vi "2 MissionHeadingGoodness.vi"(6 "Waypoint in":refnum<class "Waypoint.lvclass">, 8 "Waypoint Location":T3 {"North" format="%#_10f"; "East" format="%#_8f"}, 9 "Heading\nto Test":T2 format="%05.1f", 10 "UW Tack":dbl, 11 "Into irons?":bool) -> (0 "Pure Waypoint Goodness":dbl, 1 "Direction Change Goodness":dbl, 2 "No-Sail Goodness":dbl, 3 "Target Goodness":dbl, 4 "Pure Wind Goodness":dbl)   [LabVIEW 2011]
doc: "This VI simply takes in a heading to test, runs the necessary component goodness functions and outputs their \"goodness value\" for that heading."
uses:
  2 Typedefs/UTM Location.ctl
  2 Classes/Waypoint/Waypoint.lvclass
  2 Typedefs/heading.ctl
  2 Typedefs/apparent wind direction.ctl
  2 Globals/2 Global.vi
  2 Globals/2 TuningConstants.vi
panel:
  out "Heading Goodness":T1
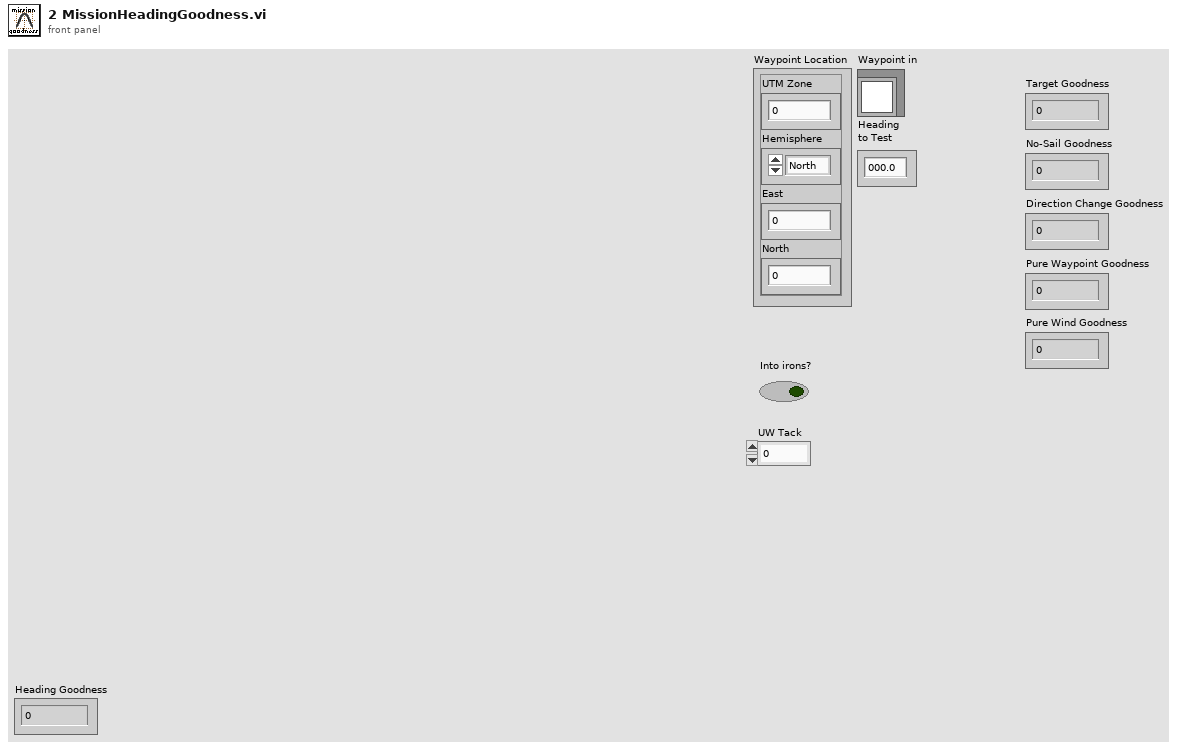
[diagram p1: front panel]
types:
  T1 = typedef "apparent wind direction.ctl" = dbl
  T2 = typedef "heading.ctl" = dbl
  T3 = typedef "UTM Location.ctl" = cluster{"UTM Zone":dbl, "Hemisphere":enum16{"North", "South"}, "East":dbl, "North":dbl}
  T4 = typedef "absolute wind direction.ctl" = dbl
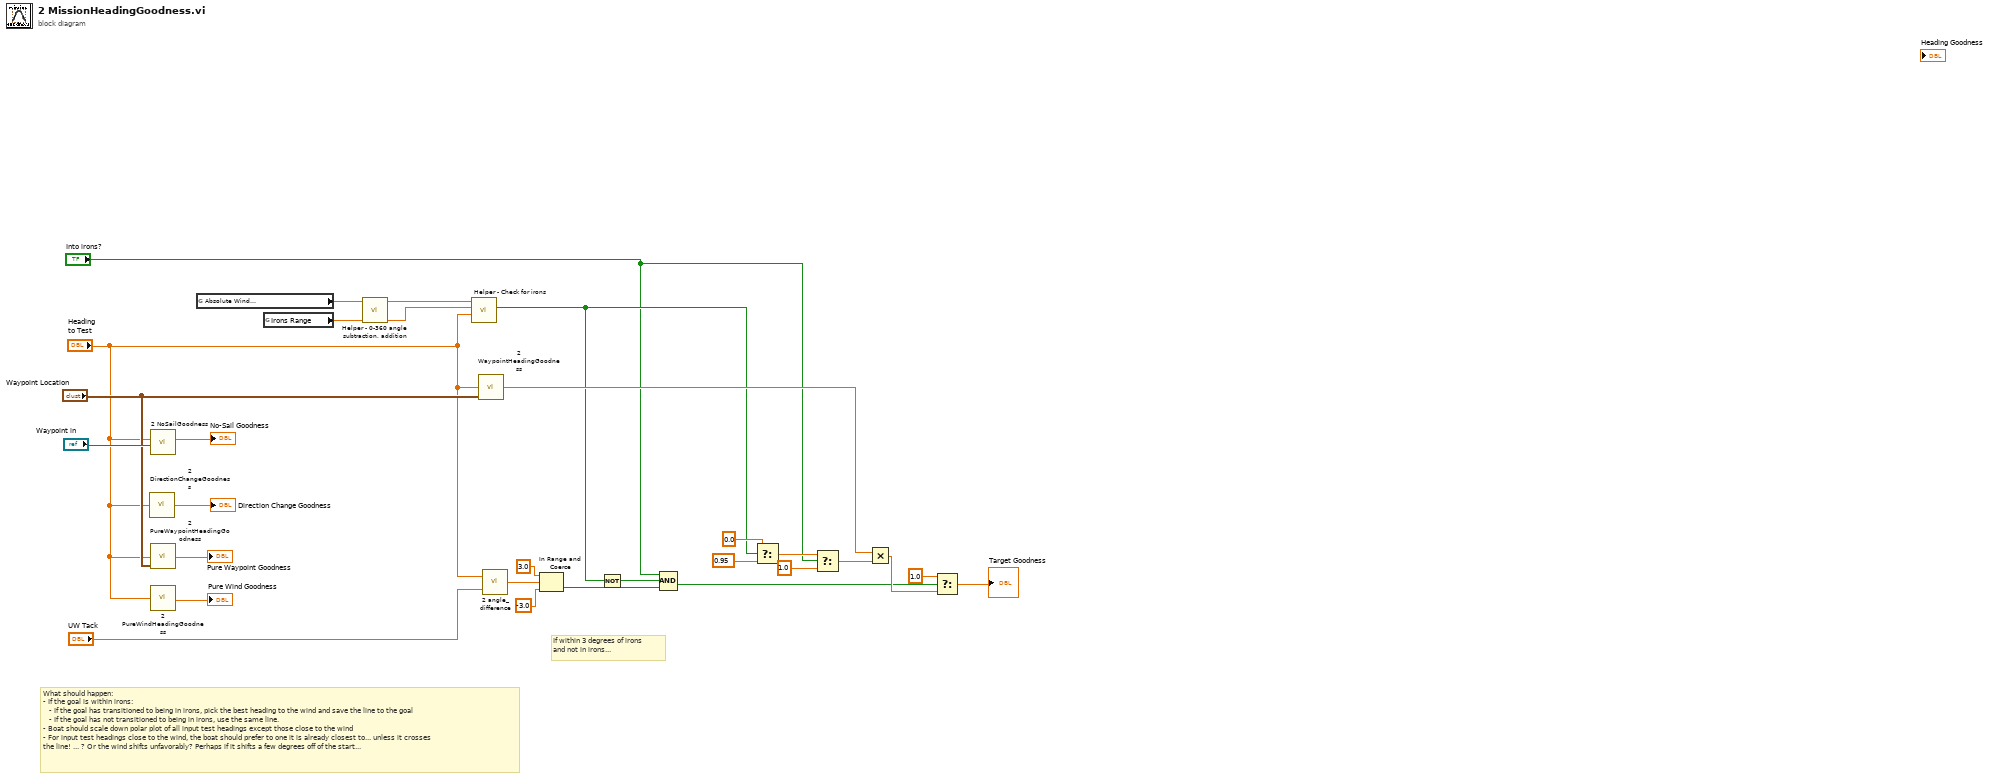
[diagram p0: block diagram]
diagram:
  # "If within 3 degrees of irons\nand not in irons..."
  # "What should happen:\n- If the goal is within irons:\n   - If the goal has transitioned to being in irons, pick the best heading to the wind and save the line to the goal\n   - If the goal has not transitioned to being in irons, use the same line.\n- Boat should scale down polar plot of all input test headings except those close to the wind\n- For input test headings close to the wind, the boat should prefer to one it is already closest to... unless it crosses\nthe line! ... ? Or the wind shifts unfavorably? Perhaps if it shifts a few degrees off of the start..."
  n1 = call "2 DirectionChangeGoodness.vi"("Test Heading"="Heading\nto Test") -> ("Goodness"=→"Direction Change Goodness":dbl)
  n2 = call "2 NoSailGoodness.vi"("Waypoint in"="Waypoint in", "Heading to Test"="Heading\nto Test") -> ("Goodness"=→"No-Sail Goodness":dbl)  [unwired: 9 in]
  n3 = call "2 PureWaypointHeadingGoodness.vi"("Waypoint Location"="Waypoint Location", "Heading to Test"="Heading\nto Test") -> ("Goodness"=→"Pure Waypoint Goodness":dbl)  [unwired: 3 in]
  n4 = call "2 PureWindHeadingGoodness.vi"("Heading\nto Test"="Heading\nto Test") -> ("Goodness"=→"Pure Wind Goodness":dbl)  [unwired: 4 in]
  n5 = global read "2 Global.vi" "Absolute Wind\nDirection (º)"() -> (w16:T4)
  n6 = global read "2 TuningConstants.vi" "Irons Range"() -> (w17:dbl)
  n7 = call "Helper - 0-360 angle subtraction, addition.vi"("y"=w17, "x"=w16) -> ("x + y"=w14:dbl, "x - y"=w15:T1)  [unwired: 8 in]
  n8 = call "Helper - Check for irons.vi"("Angle to check"="Heading\nto Test", "Wind - Irons range"=w14, "Wind + Irons range"=w15) -> ("In irons?"=w9:bool)  [unwired: 8 in]
  n9 = call "2 WaypointHeadingGoodness.vi"("Waypoint Location"="Waypoint Location", "Heading\nto Test"="Heading\nto Test") -> ("Goodness"=w10:dbl)  [unwired: 3 in]
  n10 = call "2 angle_difference.vi"("Angle 2"="UW Tack", "Angle 1"="Heading\nto Test") -> ("Difference"=w22:dbl)
  n11 = In Range and Coerce(upper limit=T1 3.0, x=w22, lower limit=T1 -3.0) -> (In Range?=w4:bool)  [unwired: 1 out]
  n12 = Not(x=w9) -> (.not. x?=w3:bool)
  n13 = Compound Arithmetic op=AND("Into irons?", w3, w4) -> (w1:bool)
  n14 = Select(t=0.0, s=w9, f=0.95 ("t")) -> (s? t:f=w12:dbl)
  n15 = Select(t=w12, s="Into irons?", f=1.0 ("t")) -> (s? t:f=w18:dbl)
  n16 = Multiply(x=w10, y=w18) -> (x*y=w6:dbl)
  n17 = Select(t=1.0, s=w1, f=w6) -> (s? t:f=→"Target Goodness":dbl)
